vi "fpga_BandPass filter_engineunit0 (M Class_50Hz).vi"(0 "input data":fxp<+/-,24,2>, 1 "ACC_Load":bool, 7 "coefficients":fxp<+/-,18,-4>[](array[numeric])=[0.0], 11 "opState":T1) -> (4 "output data":fxp<+/-,24,3>)   [LabVIEW 2013, in "NI_EP_PMU_FPGA.lvlib"]
uses:
  <vilib>/addons/Electrical Power/PMU/NI_EP_PMU_FPGA.lvlib
  <vilib>/rvi/FXPMathLib/basic elements/FxpIntAccumulator/subVIs/nifxpmath_IntAccumulator_SimConfig.ctl
  <vilib>/rvi/FXPMathLib/basic elements/FxpIntAccumulator/simVIs/DllFxpIntAccumulator_sub.vi
  <vilib>/rvi/FXPMathLib/basic elements/FxpIntAccumulator/XNode/nifxpmath_IntAccumulator.xnode
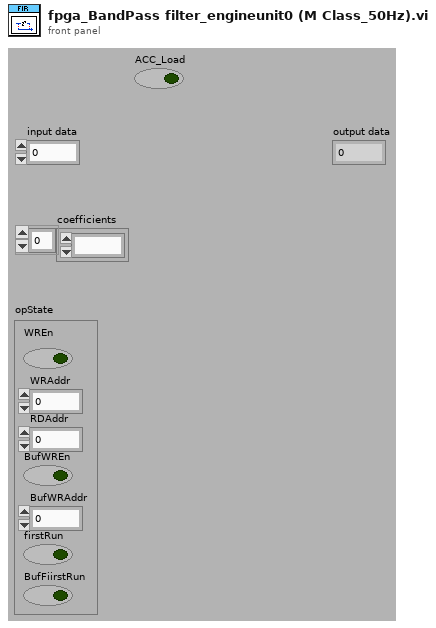
[diagram p1: front panel]
types:
  T1 = cluster{"WREn":bool, "WRAddr":fxp<+,11,11>, "RDAddr":fxp<+,11,11>, "BufWREn":bool, "BufWRAddr":fxp<+,11,11>, "firstRun":bool, "BufFiirstRun":bool}
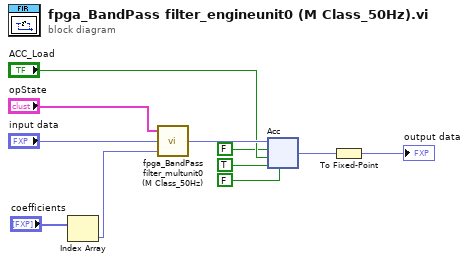
[diagram p0: block diagram]
diagram:
  n1 = Index Array ("CoefExpander")(array="coefficients") -> (element=w4:fxp<+/-,18,-4>)  [unwired: 1 in]
  n2 = call <vilib>:"fpga_BandPass filter_multunit0 (M Class_50Hz).vi"("opState"="opState", "x"="input data", "coef"=w4) -> ("y"=w11:fxp<+/-,40,3>)  [unwired: 5 in, 1 out]
  n3 = xnode ("Acc")("x"=w11, "load (F)"="ACC_Load", "is sub? (F)"=FALSE ("is sub?"), "enable (T)"=TRUE ("enable"), "carry-in/inverted borrow-in (F)"=FALSE ("carry-in/no borrow-in")) -> ("s"=w9:fxp<+/-,40,3>)  [unwired: 1 out]
  n4 = To Fixed-Point ("toOutput")(number=w9) -> (fixed-point=→"output data":fxp<+/-,24,3>)  [unwired: 1 out]
